vi "FRCts20_WebMethods_ReadData_Comment.vi"(7 "Cluster Type":T1, 8 "error in (no error)":errorcluster, 11 "httpRequestID":u32) -> (0 "error out":errorcluster, 2 "Cluster out":T1, 3 "httpRequestID out":u32)   [LabVIEW 2014, in "FRCts20_WebMethods.lvlib"]
uses:
  FRCts20_WebMethods.lvlib
  <vilib>/wsapi/NI_WebServices.lvlib
  <vilib>/regexp/Match Regular Expression.xnode
  Backend/source/VI Source/FRCts20_Backend_API/FRCts20_Backend_API_Note.ctl
  Backend/source/VI Source/FRCts20_Backend_API/FRCts20_Backend_API.lvlib
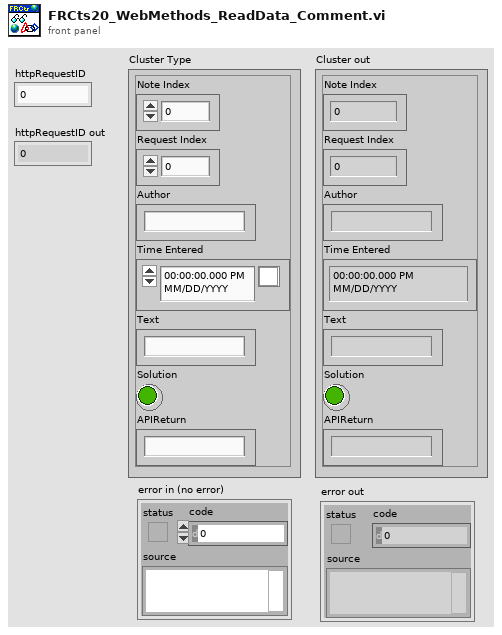
[diagram p1: front panel]
types:
  T1 = typedef "FRCts20_Backend_API.lvlib/FRCts20_Backend_API_Note.ctl" = cluster{"Note Index":u32, "Request Index":u32, "Author":string, "Time Entered":timestamp, "Text":string, "Solution":bool, "APIReturn":string}
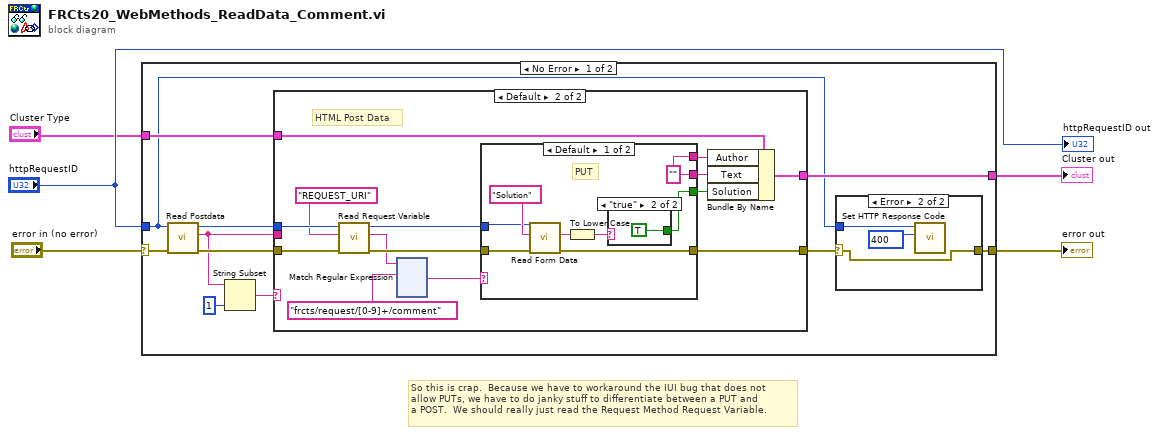
[diagram p0: block diagram]
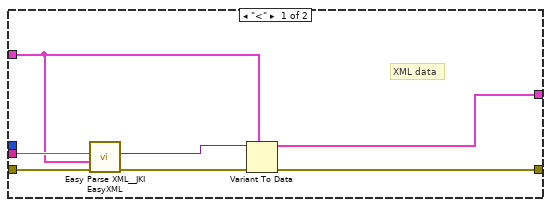
[diagram p3: hidden frame]
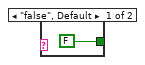
[diagram p4: hidden frame]
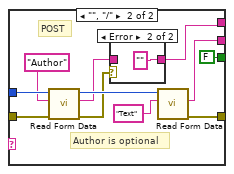
[diagram p5: hidden frame]
diagram:
  # "So this is crap.  Because we have to workaround the IUI bug that does not\nallow PUTs, we have to do janky stuff to differentiate between a PUT and \na POST.  We should really just read the Request Method Request Variable."
  n1 = case shown="No Error" "error in (no error)" {
    selector: "error in (no error)" -> [w16 w177]
    tunnel: "httpRequestID" -> [w6 _]
    tunnel: "Cluster Type" -> [w10 w176]
    tunnel: [w8 w177] -> w4
    tunnel: [w9 w176] -> w1
    frame No Error {
      n2 = call <vilib>:"Read Postdata.vi"("error in (no error)"=w16, "httpRequestID"=w6) -> ("error out"=w13:errorcluster, "postdata"=w11:string, "httpRequestID out"=w12:u32)  [unwired: 7 in]
      n3 = String Subset(string=w11, length (rest)=1 ("length (rest)")) -> (substring=w14:string)  [unwired: 1 in]
      n4 = case shown="Default" w14 {
        tunnel: w13 -> [w27 w38]
        tunnel: w12 -> [_ w37]
        tunnel: w11 -> [w26 _]
        tunnel: w10 -> [w23 w41]
        tunnel: [w21 w33] -> w7
        tunnel: [w22 w40] -> w9
        frame "<" {
          # "XML data"
          n5 = call <vilib>:"Easy Parse XML__JKI EasyXML.vi"("error in (no error)"=w27, "LabVIEW Data (Type)"=w23, "XML String"=w26) -> ("error out"=w25:errorcluster, "LabVIEW Data"=w24:variant)  [unwired: 7 in]
          n6 = Variant To Data(error in=w25, type=w23, Variant=w24) -> (data=w22:T1, error out=w21:errorcluster)
        }
        frame Default {
          # "HTML Post Data"
          n7 = call <vilib>:"Read Request Variable.vi"("error in (no error)"=w38, "variable name"="REQUEST_URI", "httpRequestID"=w37) -> ("error out"=w35:errorcluster, "value"=w30:string, "httpRequestID out"=w34:u32)  [unwired: 6 in]
          n8 = xnode "Match Regular Expression"("input string"=w30, "regular expression"="frcts/request/[0-9]+/comment") -> ("after match"=w29:string)  [unwired: 4 in, 4 out]
          n9 = case shown="Default" w29 {
            tunnel: w35 -> [w157 w173]
            tunnel: w34 -> [w156 w172]
            tunnel: [w153 w166] -> w39
            tunnel: [w154 w165] -> w33
            tunnel: [w153 w164] -> w32
            tunnel: [w155 FALSE] -> w31
            frame Default {
              w153 = "" ("value")
              # "PUT"
              n10 = call <vilib>:"Read Form Data.vi"("error in (no error)"=w157, "key"="Solution", "httpRequestID"=w156) -> ("error out"=w154:errorcluster, "value"=w158:string)  [unwired: 5 in, 2 out]
              n11 = To Lower Case(string=w158) -> (all lower case string=w159:string)
              n12 = case shown="\"true\"" w159 {
                tunnel: [FALSE TRUE] -> w155
                frame "false", Default {
                }
                frame "true" {
                }
              }
            }
            frame "", "/" {
              # "POST"
              # "Author is optional"
              n13 = call <vilib>:"Read Form Data.vi"("error in (no error)"=w173, "key"="Author", "httpRequestID"=w172) -> ("error out"=w168:errorcluster, "value"=w167:string, "httpRequestID out"=w171:u32)  [unwired: 5 in, 1 out]
              n14 = case shown="Error" w168 {
                tunnel: w167 -> [w174 _]
                tunnel: [w174 ""] -> w166
                frame No Error {
                }
                frame Error {
                }
              }
              n15 = call <vilib>:"Read Form Data.vi"("key"="Text", "httpRequestID"=w171) -> ("error out"=w165:errorcluster, "value"=w164:string)  [unwired: 6 in, 2 out]
            }
          }
          n16 = Bundle By Name(cluster=w41, "Author"=w39, "Text"=w32, "Solution"=w31) -> (w40:T1)
        }
      }
      n17 = case shown="Error" w7 {
        selector: w7 -> [w17 w18]
        tunnel: [w17 w18] -> w8
        tunnel: w6 -> [_ w20]
        frame No Error {
        }
        frame Error {
          w19 = 400 items=["100"=100, "101"=101, "200"=200, "201"=201, "202"=202, "203"=203, "204"=204, "205"=205, "206"=206, "300"=300, "301"=301, "302"=302, "303"=303, "304"=304, "305"=305, "306"=306, "307"=307, "400"=400, "401"=401, "402"=402, "403"=403, "404"=404, "405"=405, "406"=406, "407"=407, "408"=408, "409"=409, "410"=410, "411"=411, "412"=412, "413"=413, "414"=414, "415"=415, "416"=416, "417"=417, "500"=500, "501"=501, "502"=502, "503"=503, "504"=504, "505"=505] ("response code (200)")
          n18 = call <vilib>:"Set HTTP Response Code.vi"("response code (200)"=w19, "httpRequestID"=w20) -> ()  [unwired: 8 in, 2 out]
        }
      }
    }
    frame Error {
    }
  }
  "error out" <- w4
  "Cluster out" <- w1
  "httpRequestID out" <- "httpRequestID"
